vi "Clear Data2.vi"(8 "error in (no error)":errorcluster, 9 "Time":u32, 11 "Data In":T1) -> (0 "error out":errorcluster, 3 "Data out":T1)   [LabVIEW 2014]
uses:
  controls/Data1.ctl
  controls/Payjson.ctl
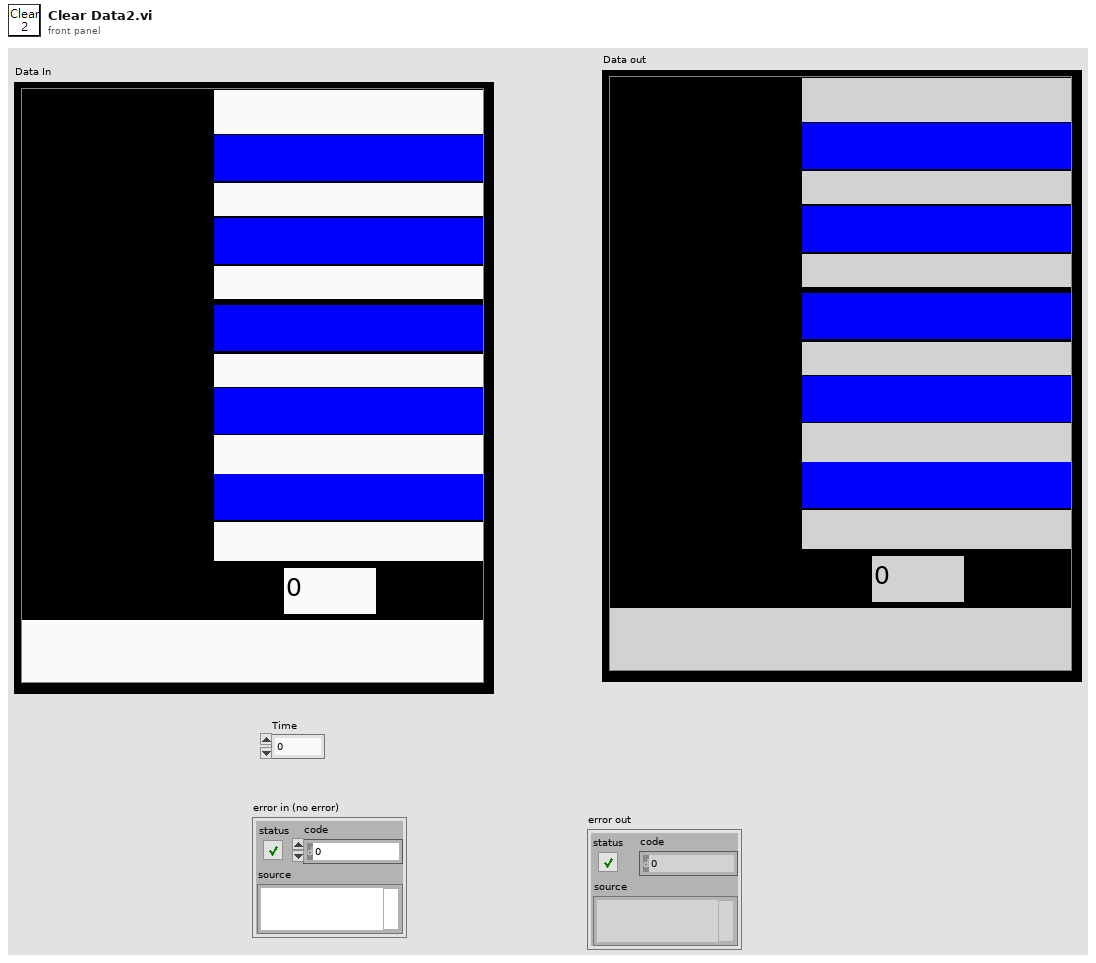
[diagram p1: front panel]
types:
  T1 = typedef "Data1.ctl" = cluster{"Date":string, "BarCode1":string, "BarCode2":string, "BarCode3":string, "Message":string, "OK Count":u16, "NG Count":u16, "Total Count":u16, "ModelData":string[][], "OK&NG":bool, "COM1":refnum<visa-resource-name>, "COM2":refnum<visa-resource-name>, "IO":i32, "Time":u32, "TCP":refnum<k5>, "TCP 2":refnum<k5>, "COM1 2":refnum<visa-resource-name>, "CheckNum":string, "BarCode1_1":string, "BarCode2_1":string, "BarCode3_1":string, "日期":string, "機種":string, "機號":string, "商品條碼1":string, "OK_1":string, "OK":string, "NG":string, "NG_1":string, "Total":string, "Total_1":string, "ClaerTime":u32, "Pjson":T2, "LotNo":string[], "CheckParsArray":string[], "BarCode4":string, "BarCode4_1":string, "商品條碼2":string, "BarCode5":string, "BarCode5_1":string, "商品條碼3":string, "ReScanNG":i32, "NGTimeCT":u32}
  T2 = typedef "Payjson.ctl" = cluster{"DEPT":string, "LINE":string, "STANO":string, "WORKNO":string, "PRODSN":string, "COMPNTID":string, "COMPNTLOT":string, "COMPNTSN":string, "USEDQTY":i16, "OPDATE":string, "OPUSER":string, "RECVDATE":string, "MMODU":string}[]
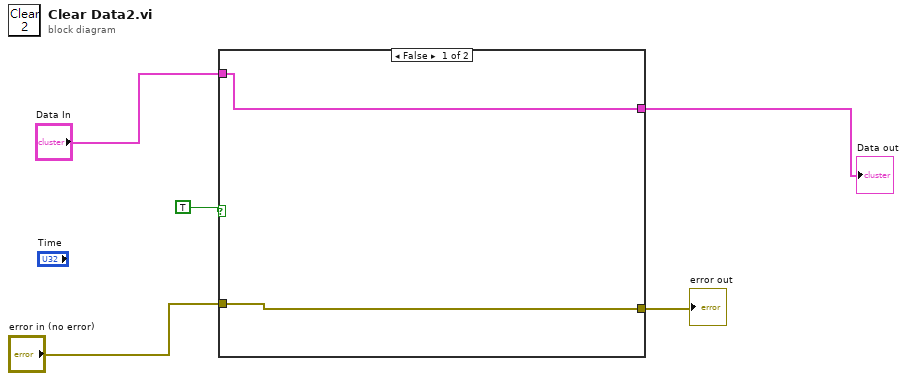
[diagram p0: block diagram]
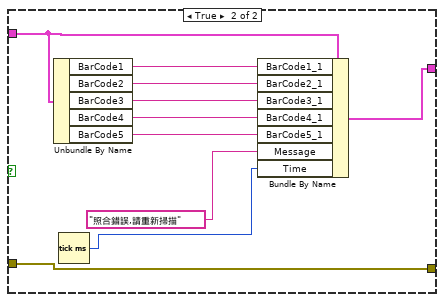
[diagram p2: hidden frame]
diagram:
  n1 = case shown="False" TRUE {
    tunnel: [w6 w16] -> w1
    tunnel: "error in (no error)" -> [w7 w17]
    tunnel: [w7 w17] -> w4
    tunnel: "Data In" -> [w6 w13]
    frame False {
    }
    frame True {
      n2 = Unbundle By Name(w13) -> ("BarCode1"=w12:string, "BarCode2"=w11:string, "BarCode3"=w10:string, "BarCode4"=w9:string, "BarCode5"=w8:string)
      n3 = Tick Count (ms)() -> (millisecond timer value=w14:u32)
      n4 = Bundle By Name(cluster=w13, "BarCode1_1"=w12, "BarCode2_1"=w11, "BarCode3_1"=w10, "BarCode4_1"=w9, "BarCode5_1"=w8, "Message"="照合錯誤,請重新掃描", "Time"=w14) -> (w16:T1)
    }
  }
  "error out" <- w4
  "Data out" <- w1
